vi "Main.vi"() -> ()   [LabVIEW 2019]
uses:
  <vilib>/sound2/lvsound2.llb/Sound Data Format.ctl
  <vilib>/sound2/lvsound2.llb/Sampling Mode.ctl
  <vilib>/sound2/lvsound2.llb/Sound Input Read (DBL).vi
panel:
  out "Threshold Exceeded?":bool
  in  "Type":T1(ring)
  in  "Order":i32=6
  in  "Lower Fc":dbl=300.0 format="%#_13g"
  in  "Upper Fc":dbl=3500.0 format="%#_13g"
  in  "Threshold, dB":dbl=-100.0 format="%#_13g"
  out "Spectrum Data":cluster{"f0":dbl, "df":dbl, "magnitude":dbl[]}[](graph)
  out "Raw Data":waveform(dbl)[](graph)
  # "FILTER SETTINGS"
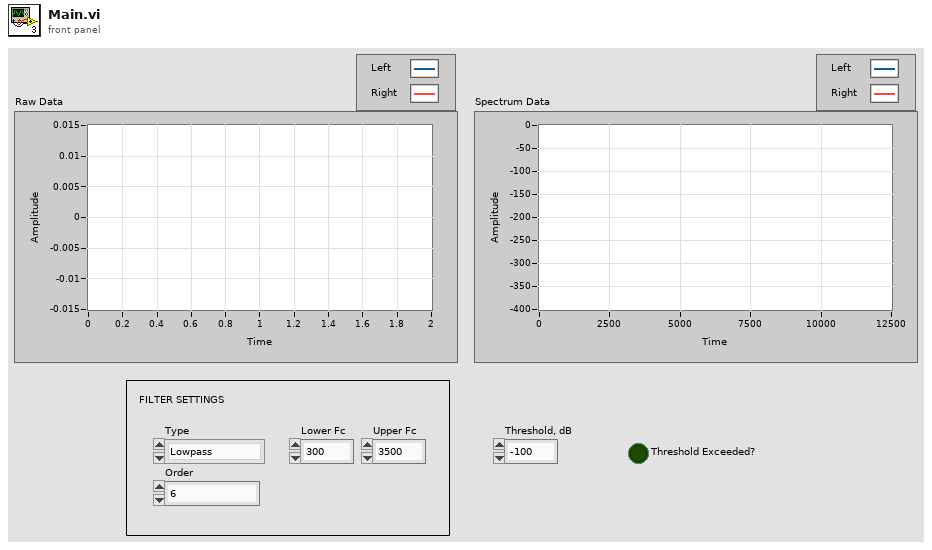
[diagram p1: front panel]
types:
  T1 = enum16{"Lowpass", "Highpass", "Bandpass", "Bandstop"}
  T2 = cluster{"Topology":enum16{"Off", "Butterworth", "Chebyshev", "Inverse Chebyshev", "Elliptic", "Bessel"}, "Type":enum16{"Lowpass", "Highpass", "Bandpass", "Bandstop"}, "Order":i32, "Lower Fc":dbl, "Upper Fc":dbl, "PB Ripple":dbl, "SB Attenuation":dbl}
  T3 = typedef "Sampling Mode.ctl" = i32
  T4 = typedef "Sound Data Format.ctl" = cluster{"sample rate (S/s)":dbl, "number of channels":i32, "bits per sample":i32}
  T5 = typedef "Sound Input Task ID.ctl" = u32
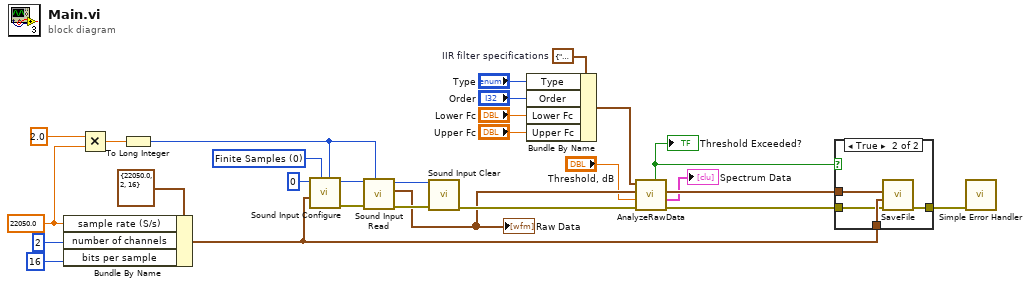
[diagram p0: block diagram]
diagram:
  w2 = T2 {"Topology"=enum."Butterworth", "Type"=enum."Lowpass", "Order"=1, "Lower Fc"=100.0, "Upper Fc"=200.0, "PB Ripple"=1.0, "SB Attenuation"=60.0}  # IIR filter specifications
  w21 = T3 0 items=["Finite Samples", "Continuous Samples"] ("sample mode")
  w15 = 22050.0 ("Sample rate (Hz)")
  n1 = Bundle By Name(cluster=T4 {"sample rate (S/s)"=22050.0, "number of channels"=2, "bits per sample"=16} ("Sound Format"), "sample rate (S/s)"=w15, "number of channels"=2 ("#Channels"), "bits per sample"=16 ("Resolution (bits)")) -> (w14:T4)
  n2 = Multiply(x=2.0 ("Duration (s)"), y=w15) -> (x*y=w19:dbl)
  n3 = To Long Integer(number=w19) -> (32bit integer=w18:i32)
  n4 = call <vilib>:"Sound Input Configure.vi"("number of samples/ch"=w18, "sample mode"=w21, "sound format"=w14, "device ID"=u32 0 ("Device")) -> ("error out"=w24:errorcluster, "task ID"=w20:T5)  [unwired: 6 in]
  n5 = call-poly <vilib>:"Sound Input Read.vi"("number of samples/ch"=w18, "error in (no error)"=w24, "task ID"=w20) -> ("error out"=w16:errorcluster, "data"=w12:waveform(dbl)[], "task ID out"=w17:T5)  [unwired: 6 in]
  "Raw Data" <- w12
  n6 = call <vilib>:"Sound Input Clear.vi"("error in (no error)"=w16, "task ID"=w17) -> ("error out"=w13:errorcluster)  [unwired: 9 in]
  n7 = Bundle By Name(cluster=w2, "Type"="Type", "Order"="Order", "Lower Fc"="Lower Fc", "Upper Fc"="Upper Fc") -> (w3:T2)
  n8 = call "AnalyzeRawData.vi"("error in (no error)"=w13, "Threshold, dB"="Threshold, dB", "Raw Data"=w12, "IIR Filter Specifications"=w3) -> ("error out"=w9:errorcluster, "Power Spectrum / PSD"=→"Spectrum Data":cluster{"f0":dbl, "df":dbl, "magnitude":dbl[]}[], "Filtered Data"=w11:waveform(dbl)[], "Threshold Exceeded?"=w1:bool)  [unwired: 4 in]
  "Threshold Exceeded?" <- w1
  n9 = case shown="True" w1 {
    tunnel: [w29 w33] -> w25
    tunnel: w14 -> [_ w32]
    tunnel: w9 -> [w29 w31]
    tunnel: w11 -> [_ w30]
    frame False {
    }
    frame True {
      n10 = call "SaveFile.vi"("error in (no error)"=w31, "Sound Format"=w32, "Waveform(s) in"=w30) -> ("error out"=w33:errorcluster)  [unwired: 8 in]
    }
  }
  n11 = call <vilib>:"Simple Error Handler.vi"("error in (no error)"=w25) -> ()  [unwired: 4 in, 5 out]
